vi "Run.vi"(8 "error in (no error)":errorcluster, 11 "Channel GUI in":refnum<class "Channel GEI.lvclass">) -> (0 "error out":errorcluster, 3 "Channel GUI out":refnum<class "Channel GEI.lvclass">)   [LabVIEW 2018, in "Channel GEI.lvclass"]
uses:
  Channel GEI.lvclass
  Channel GEI.lvclass/Channel GEI.ctl
  Interface/Interface.lvclass/Interface.ctl
  State Machine/State Machine.lvclass
  RxTx/RxTx.lvclass
  Interface/Interface.lvclass
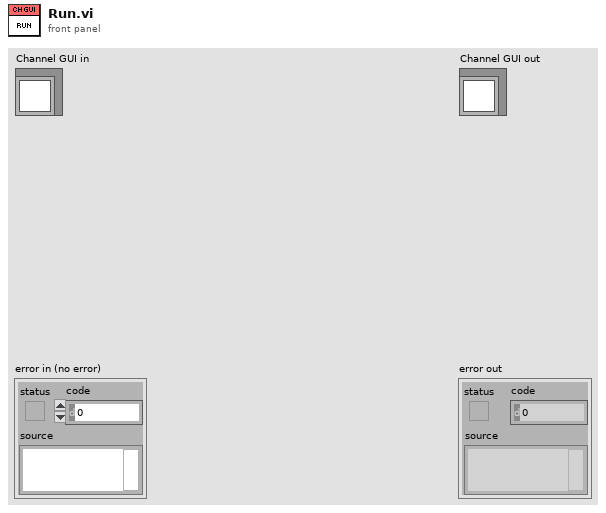
[diagram p1: front panel]
types:
  T1 = cluster{"COOLER_POWER_STATUS":u16, "TEMP":i32, "EXPTIME":dbl, "#FRAMES":u32, "#CUBES":u32}
  T2 = cluster{"CUBE_EXPOSURE_TIME":sgl, "CUBES_DONE":u16, "LAST_IMAGE_NAME":string, "DISK_SPACE":u16, "FRAMES_DONE":u16, "CCD_STATUS":string, "CURRENT_TEMPERATURE":i16, "TEMPERATURE_STATUS":string, "FRAME_EXPOSURE_TIME":u16, "CCD_ON_OFF":bool, "SERIAL_NUMBER":u16, "ACQUIRING":bool}
  T3 = cluster{"PREAMP":u16, "READOUT_RATE":u16, "EM_GAIN":u16, "VBIN":u16, "INITIAL_LINE":u16, "INITIAL_COLUMN":u16, "FINAL_LINE":u16, "FINAL_COLUMN":u16, "TRIGGER_MODE":u16, "HBIN":u16, "SHUTTER_TTL":u16, "SHUTTER_MODE":u16, "SHUTTER_OPENING_TIME":u16, "SHUTTER_CLOSING_TIME":u16, "VERTICAL_SHIFT_SPEED":u16, "READ_MODE":u16, "FRAME_TRANSFER":bool, "VERTICAL_CLOCK_VOLTAGE":u16, "ACQUISITION_MODE":u16, "AD_CHANNEL":u16, "EM_MODE":u16}
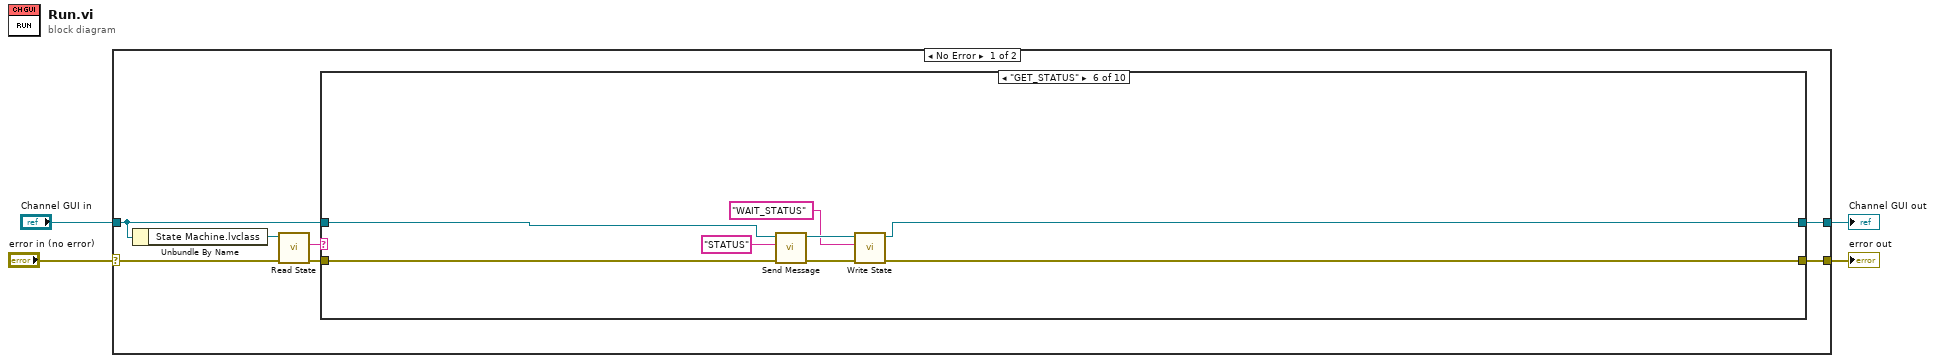
[diagram p0: block diagram]
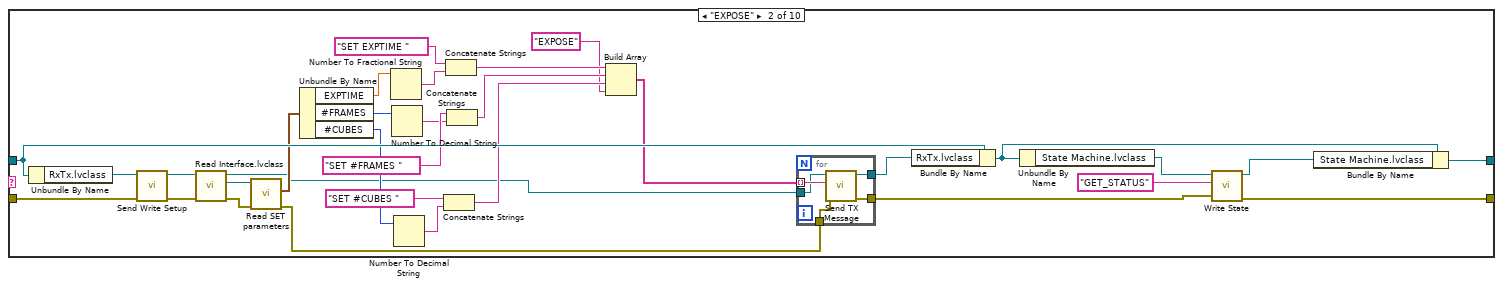
[diagram p3: hidden frame]
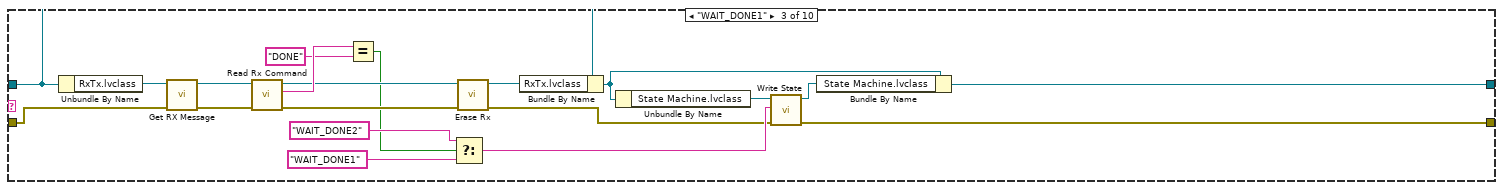
[diagram p4: hidden frame]
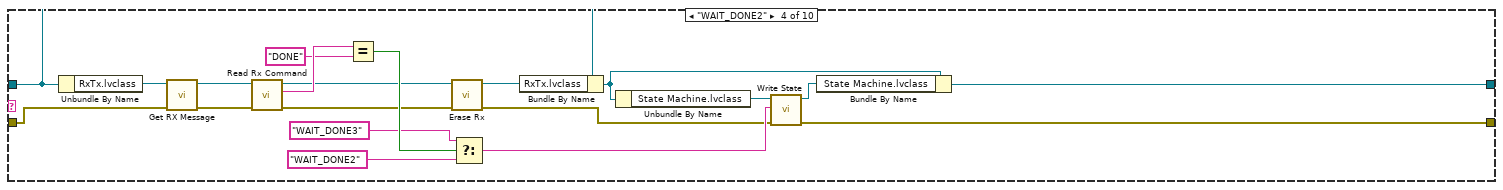
[diagram p5: hidden frame]
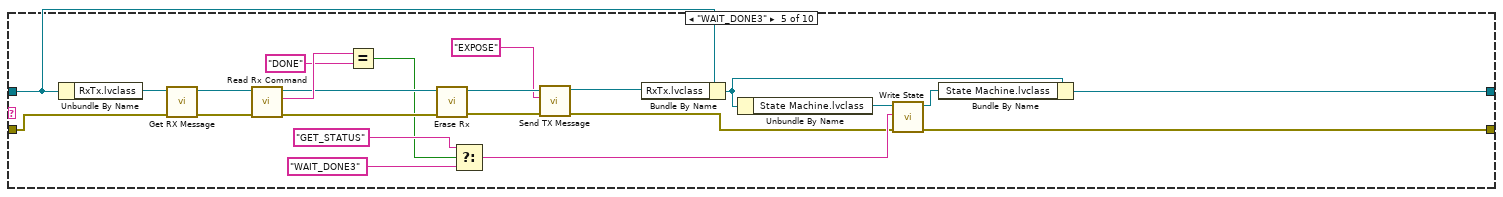
[diagram p6: hidden frame]
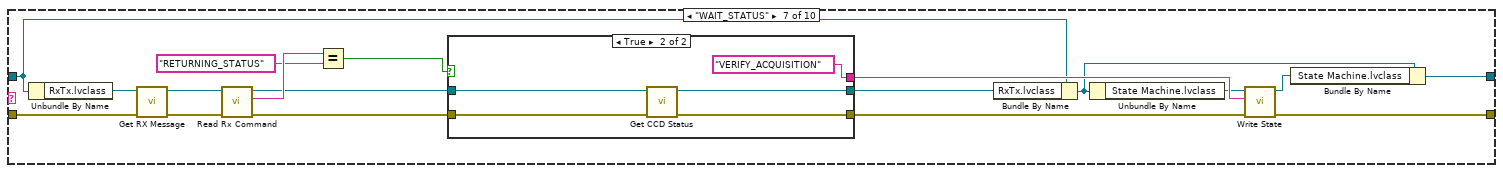
[diagram p7: hidden frame]
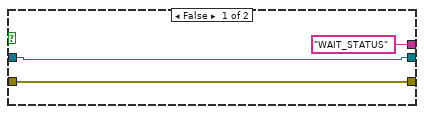
[diagram p8: hidden frame]
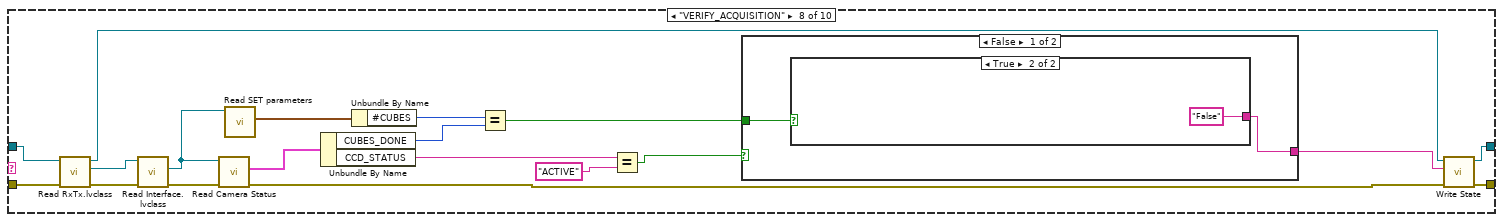
[diagram p9: hidden frame]
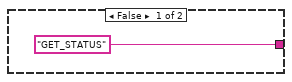
[diagram p10: hidden frame]
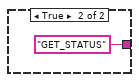
[diagram p11: hidden frame]
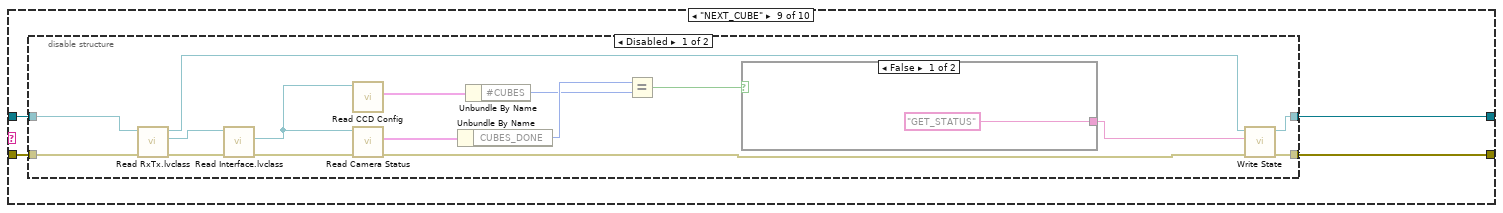
[diagram p12: hidden frame]
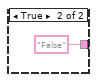
[diagram p13: hidden frame]
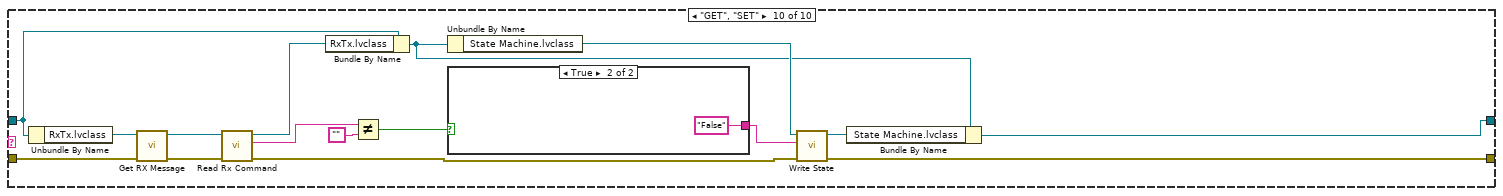
[diagram p15: hidden frame]
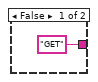
[diagram p16: hidden frame]
diagram:
  n1 = case shown="No Error" "error in (no error)" {
    selector: "error in (no error)" -> [w9 w215]
    tunnel: [w11 w215] -> w2
    tunnel: "Channel GUI in" -> [w7 w214]
    tunnel: [w6 w214] -> w1
    frame No Error {
      n2 = Unbundle By Name(w7) -> ("State Machine.lvclass"=w10:refnum<class "State Machine.lvclass">)
      n3 = call-dynamic "Read State.vi"("error in (no error)"=w9, "State Machine in"=w10) -> ("error out"=w8:errorcluster, "State"=w5:string)  [unwired: 7 in, 1 out]
      n4 = case shown="\"GET_STATUS\"" w5 {
        tunnel: w8 -> [w13 w37 w65 w85 w108 w121 w136 w159 w172 w208]
        tunnel: [w13 w41 w61 w81 w104 w116 w139 w165 w174 w211] -> w11
        tunnel: w7 -> [w12 w43 w60 w80 w103 w114 w125 w160 w173 w200]
        tunnel: [w12 w42 w62 w82 w105 w117 w123 w166 w175 w198] -> w6
        frame "False", Default {
        }
        frame "EXPOSE" {
          n5 = Unbundle By Name(w43) -> ("RxTx.lvclass"=w38:refnum<class "RxTx.lvclass">)
          n6 = call "Send Write Setup.vi"("error in (no error)"=w37, "RxTx in"=w38) -> ("error out"=w33:errorcluster, "RxTx out"=w34:refnum<class "RxTx.lvclass">)  [unwired: 8 in]
          n7 = call "Read Interface.lvclass.vi"("error in (no error)"=w33, "RxTx in"=w34) -> ("error out"=w31:errorcluster, "Interface.lvclass"=w32:refnum<class "Interface.lvclass">, "RxTx out"=w16:refnum<class "RxTx.lvclass">)  [unwired: 7 in]
          n8 = call "Read SET parameters.vi"("error in (no error)"=w31, "Interface in"=w32) -> ("error out"=w15:errorcluster, "SET parameters"=w29:T1)  [unwired: 7 in, 1 out]
          n9 = Unbundle By Name(w29) -> ("EXPTIME"=w28:dbl, "#FRAMES"=w26:u32, "#CUBES"=w21:u32)
          n10 = Number To Fractional String(number=w28) -> (F-format string=w30:string)  [unwired: 3 in]
          n11 = Number To Decimal String(number=w26) -> (decimal integer string=w24:string)  [unwired: 1 in]
          n12 = Number To Decimal String(number=w21) -> (decimal integer string=w22:string)  [unwired: 1 in]
          n13 = Concatenate Strings("SET #CUBES ", w22) -> (w18:string)
          n14 = Concatenate Strings("SET EXPTIME ", w30) -> (w20:string)
          n15 = Concatenate Strings("SET #FRAMES ", w24) -> (w19:string)
          n16 = Build Array(w20, w19, w18, "EXPOSE") -> (w17:string[])
          n17 = for {
            tunnel: [w50] -> w36
            tunnel: [w49] -> w35
            tunnel: w17 -> [w48] mode=indexing
            tunnel: w16 -> [w47]
            tunnel: w15 -> [w46]
            n18 = call "Send TX Message.vi"("error in (no error)"=w46, "element"=w48, "RxTx in"=w47) -> ("error out"=w50:errorcluster, "RxTx out"=w49:refnum<class "RxTx.lvclass">)  [unwired: 7 in]
          }
          n19 = Bundle By Name(cluster=w43, "RxTx.lvclass"=w35) -> (w44:refnum<class "Channel GEI.lvclass">)
          n20 = Unbundle By Name(w44) -> ("State Machine.lvclass"=w45:refnum<class "State Machine.lvclass">)
          n21 = call-dynamic "Write State.vi"("error in (no error)"=w36, "State"="GET_STATUS" ("New_State"), "State Machine in"=w45) -> ("error out"=w41:errorcluster, "State Machine out"=w40:refnum<class "State Machine.lvclass">)  [unwired: 7 in]
          n22 = Bundle By Name(cluster=w44, "State Machine.lvclass"=w40) -> (w42:refnum<class "Channel GEI.lvclass">)
        }
        frame "WAIT_DONE1" {
          n23 = Unbundle By Name(w60) -> ("RxTx.lvclass"=w70:refnum<class "RxTx.lvclass">)
          n24 = call "Get RX Message.vi"("error in (no error)"=w65, "RxTx in"=w70) -> ("error out"=w69:errorcluster, "RxTx out"=w68:refnum<class "RxTx.lvclass">)  [unwired: 8 in]
          n25 = call "Read Rx Command.vi"("error in (no error)"=w69, "RxTx in"=w68) -> ("error out"=w53:errorcluster, "Rx Command"=w67:string, "RxTx out"=w52:refnum<class "RxTx.lvclass">)  [unwired: 7 in]
          n26 = Equal?(x=w67, y="DONE") -> (x = y?=w51:bool)
          n27 = Select(t="WAIT_DONE2", s=w51, f="WAIT_DONE1") -> (s? t:f=w56:string)
          n28 = call "Erase Rx.vi"("error in (no error)"=w53, "RxTx in"=w52) -> ("error out"=w54:errorcluster, "RxTx out"=w55:refnum<class "RxTx.lvclass">)  [unwired: 8 in]
          n29 = Bundle By Name(cluster=w60, "RxTx.lvclass"=w55) -> (w63:refnum<class "Channel GEI.lvclass">)
          n30 = Unbundle By Name(w63) -> ("State Machine.lvclass"=w59:refnum<class "State Machine.lvclass">)
          n31 = call-dynamic "Write State.vi"("error in (no error)"=w54, "State"=w56, "State Machine in"=w59) -> ("error out"=w61:errorcluster, "State Machine out"=w64:refnum<class "State Machine.lvclass">)  [unwired: 7 in]
          n32 = Bundle By Name(cluster=w63, "State Machine.lvclass"=w64) -> (w62:refnum<class "Channel GEI.lvclass">)
        }
        frame "WAIT_DONE2" {
          n33 = Unbundle By Name(w80) -> ("RxTx.lvclass"=w90:refnum<class "RxTx.lvclass">)
          n34 = call "Get RX Message.vi"("error in (no error)"=w85, "RxTx in"=w90) -> ("error out"=w89:errorcluster, "RxTx out"=w88:refnum<class "RxTx.lvclass">)  [unwired: 8 in]
          n35 = call "Read Rx Command.vi"("error in (no error)"=w89, "RxTx in"=w88) -> ("error out"=w71:errorcluster, "Rx Command"=w87:string, "RxTx out"=w72:refnum<class "RxTx.lvclass">)  [unwired: 7 in]
          n36 = Equal?(x=w87, y="DONE") -> (x = y?=w78:bool)
          n37 = call "Erase Rx.vi"("error in (no error)"=w71, "RxTx in"=w72) -> ("error out"=w73:errorcluster, "RxTx out"=w74:refnum<class "RxTx.lvclass">)  [unwired: 8 in]
          n38 = Select(t="WAIT_DONE3", s=w78, f="WAIT_DONE2") -> (s? t:f=w75:string)
          n39 = Bundle By Name(cluster=w80, "RxTx.lvclass"=w74) -> (w83:refnum<class "Channel GEI.lvclass">)
          n40 = Unbundle By Name(w83) -> ("State Machine.lvclass"=w79:refnum<class "State Machine.lvclass">)
          n41 = call-dynamic "Write State.vi"("error in (no error)"=w73, "State"=w75, "State Machine in"=w79) -> ("error out"=w81:errorcluster, "State Machine out"=w84:refnum<class "State Machine.lvclass">)  [unwired: 7 in]
          n42 = Bundle By Name(cluster=w83, "State Machine.lvclass"=w84) -> (w82:refnum<class "Channel GEI.lvclass">)
        }
        frame "WAIT_DONE3" {
          n43 = Unbundle By Name(w103) -> ("RxTx.lvclass"=w113:refnum<class "RxTx.lvclass">)
          n44 = call "Get RX Message.vi"("error in (no error)"=w108, "RxTx in"=w113) -> ("error out"=w112:errorcluster, "RxTx out"=w111:refnum<class "RxTx.lvclass">)  [unwired: 8 in]
          n45 = call "Read Rx Command.vi"("error in (no error)"=w112, "RxTx in"=w111) -> ("error out"=w97:errorcluster, "Rx Command"=w110:string, "RxTx out"=w98:refnum<class "RxTx.lvclass">)  [unwired: 7 in]
          n46 = Equal?(x=w110, y="DONE") -> (x = y?=w96:bool)
          n47 = call "Erase Rx.vi"("error in (no error)"=w97, "RxTx in"=w98) -> ("error out"=w92:errorcluster, "RxTx out"=w95:refnum<class "RxTx.lvclass">)  [unwired: 8 in]
          n48 = Select(t="GET_STATUS", s=w96, f="WAIT_DONE3") -> (s? t:f=w99:string)
          n49 = call "Send TX Message.vi"("error in (no error)"=w92, "element"="EXPOSE", "RxTx in"=w95) -> ("error out"=w93:errorcluster, "RxTx out"=w94:refnum<class "RxTx.lvclass">)  [unwired: 7 in]
          n50 = Bundle By Name(cluster=w103, "RxTx.lvclass"=w94) -> (w106:refnum<class "Channel GEI.lvclass">)
          n51 = Unbundle By Name(w106) -> ("State Machine.lvclass"=w102:refnum<class "State Machine.lvclass">)
          n52 = call-dynamic "Write State.vi"("error in (no error)"=w93, "State"=w99, "State Machine in"=w102) -> ("error out"=w104:errorcluster, "State Machine out"=w107:refnum<class "State Machine.lvclass">)  [unwired: 7 in]
          n53 = Bundle By Name(cluster=w106, "State Machine.lvclass"=w107) -> (w105:refnum<class "Channel GEI.lvclass">)
        }
        frame "GET_STATUS" {
          n54 = call "Send Message.vi"("error in (no error)"=w121, "Message"="STATUS", "Channel GUI in"=w114) -> ("error out"=w119:errorcluster, "Channel GUI out"=w118:refnum<class "Channel GEI.lvclass">)  [unwired: 7 in]
          n55 = call "Write State.vi"("error in (no error)"=w119, "State"="WAIT_STATUS" ("Message"), "Channel GEI in"=w118) -> ("error out"=w116:errorcluster, "Channel GEI out"=w117:refnum<class "Channel GEI.lvclass">)  [unwired: 7 in]
        }
        frame "WAIT_STATUS" {
          n56 = Unbundle By Name(w125) -> ("RxTx.lvclass"=w137:refnum<class "RxTx.lvclass">)
          n57 = call "Get RX Message.vi"("error in (no error)"=w136, "RxTx in"=w137) -> ("error out"=w135:errorcluster, "RxTx out"=w134:refnum<class "RxTx.lvclass">)  [unwired: 8 in]
          n58 = call "Read Rx Command.vi"("error in (no error)"=w135, "RxTx in"=w134) -> ("error out"=w130:errorcluster, "Rx Command"=w131:string, "RxTx out"=w129:refnum<class "RxTx.lvclass">)  [unwired: 7 in]
          n59 = Equal?(x=w131, y="RETURNING_STATUS") -> (x = y?=w132:bool)
          n60 = case shown="True" w132 {
            tunnel: ["WAIT_STATUS" "VERIFY_ACQUISITION"] -> w133
            tunnel: w130 -> [w140 w146]
            tunnel: w129 -> [w141 w145]
            tunnel: [w140 w144] -> w128
            tunnel: [w141 w143] -> w127
            frame False {
            }
            frame True {
              n61 = call "Get CCD Status.vi"("error in (no error)"=w146, "RxTx in"=w145) -> ("error out"=w144:errorcluster, "RxTx out"=w143:refnum<class "RxTx.lvclass">)  [unwired: 8 in]
            }
          }
          n62 = Bundle By Name(cluster=w125, "RxTx.lvclass"=w127) -> (w124:refnum<class "Channel GEI.lvclass">)
          n63 = Unbundle By Name(w124) -> ("State Machine.lvclass"=w126:refnum<class "State Machine.lvclass">)
          n64 = call-dynamic "Write State.vi"("error in (no error)"=w128, "State"=w133, "State Machine in"=w126) -> ("error out"=w139:errorcluster, "State Machine out"=w138:refnum<class "State Machine.lvclass">)  [unwired: 7 in]
          n65 = Bundle By Name(cluster=w124, "State Machine.lvclass"=w138) -> (w123:refnum<class "Channel GEI.lvclass">)
        }
        frame "VERIFY_ACQUISITION" {
          n66 = call "Read RxTx.lvclass.vi"("error in (no error)"=w159, "Channel GUI in"=w160) -> ("error out"=w163:errorcluster, "RxTx.lvclass"=w161:refnum<class "RxTx.lvclass">, "Channel GUI out"=w154:refnum<class "Channel GEI.lvclass">)  [unwired: 7 in]
          n67 = call "Read Interface.lvclass.vi"("error in (no error)"=w163, "RxTx in"=w161) -> ("error out"=w162:errorcluster, "Interface.lvclass"=w150:refnum<class "Interface.lvclass">)  [unwired: 7 in, 1 out]
          n68 = call "Read Camera Status.vi"("error in (no error)"=w162, "Interface in"=w150) -> ("error out"=w153:errorcluster, "Camera Status"=w158:T2)  [unwired: 7 in, 1 out]
          n69 = call "Read SET parameters.vi"("Interface in"=w150) -> ("SET parameters"=w149:T1)  [unwired: 8 in, 2 out]
          n70 = Unbundle By Name(w158) -> ("CUBES_DONE"=w152:u16, "CCD_STATUS"=w157:string)
          n71 = Unbundle By Name(w149) -> ("#CUBES"=w148:u32)
          n72 = Equal?(x=w148, y=w152) -> (x = y?=w151:bool)
          n73 = Equal?(x=w157, y="ACTIVE" ("Message")) -> (x = y?=w155:bool)
          n74 = case shown="False" w155 {
            tunnel: [w168 "GET_STATUS" ("Message")] -> w164
            tunnel: w151 -> [w167 _]
            frame False {
              n75 = case shown="True" w167 {
                tunnel: ["GET_STATUS" ("Message") "False" ("Message")] -> w168
                frame False {
                }
                frame True {
                }
              }
            }
            frame True {
            }
          }
          n76 = call "Write State.vi"("error in (no error)"=w153, "State"=w164, "Channel GEI in"=w154) -> ("error out"=w165:errorcluster, "Channel GEI out"=w166:refnum<class "Channel GEI.lvclass">)  [unwired: 7 in]
        }
        frame "NEXT_CUBE" {
          n77 = disable-structure shown="Disabled" {
            disable-tunnel: [w191 w195] -> w175
            disable-tunnel: [w190 w194] -> w174
            disable-tunnel: w173 -> [w185 w195]
            disable-tunnel: w172 -> [w184 w194]
            frame Disabled {
              n78 = call "Read RxTx.lvclass.vi"("error in (no error)"=w184, "Channel GUI in"=w185) -> ("error out"=w188:errorcluster, "RxTx.lvclass"=w186:refnum<class "RxTx.lvclass">, "Channel GUI out"=w180:refnum<class "Channel GEI.lvclass">)  [unwired: 7 in]
              n79 = call "Read Interface.lvclass.vi"("error in (no error)"=w188, "RxTx in"=w186) -> ("error out"=w187:errorcluster, "Interface.lvclass"=w178:refnum<class "Interface.lvclass">)  [unwired: 7 in, 1 out]
              n80 = call "Read CCD Config.vi"("Interface in"=w178) -> ("Previous CCD Config"=w177:T3)  [unwired: 8 in, 2 out]
              n81 = call "Read Camera Status.vi"("error in (no error)"=w187, "Interface in"=w178) -> ("error out"=w179:errorcluster, "Camera Status"=w183:T2)  [unwired: 7 in, 1 out]
              n82 = Unbundle By Name(w183) -> ("CUBES_DONE"=w182:u16)
              n83 = Unbundle By Name(w177) -> ("#CUBES"=w176:u32)
              n84 = Equal?(x=w182, y=w176) -> (x = y?=w181:bool)
              n85 = case shown="False" w181 {
                tunnel: ["GET_STATUS" ("Message") "False" ("Message")] -> w189
                frame False {
                }
                frame True {
                }
              }
              n86 = call "Write State.vi"("error in (no error)"=w179, "State"=w189, "Channel GEI in"=w180) -> ("error out"=w190:errorcluster, "Channel GEI out"=w191:refnum<class "Channel GEI.lvclass">)  [unwired: 7 in]
            }
            frame Enabled {
            }
          }
        }
        frame "GET", "SET" {
          n87 = Unbundle By Name(w200) -> ("RxTx.lvclass"=w209:refnum<class "RxTx.lvclass">)
          n88 = call "Get RX Message.vi"("error in (no error)"=w208, "RxTx in"=w209) -> ("error out"=w207:errorcluster, "RxTx out"=w206:refnum<class "RxTx.lvclass">)  [unwired: 8 in]
          n89 = call "Read Rx Command.vi"("error in (no error)"=w207, "RxTx in"=w206) -> ("error out"=w196:errorcluster, "Rx Command"=w202:string, "RxTx out"=w197:refnum<class "RxTx.lvclass">)  [unwired: 7 in]
          n90 = Bundle By Name(cluster=w200, "RxTx.lvclass"=w197) -> (w199:refnum<class "Channel GEI.lvclass">)
          n91 = Not Equal?(x=w202, y="") -> (x != y?=w204:bool)
          n92 = Unbundle By Name(w199) -> ("State Machine.lvclass"=w201:refnum<class "State Machine.lvclass">)
          n93 = case shown="True" w204 {
            tunnel: ["GET" "False"] -> w205
            frame False {
            }
            frame True {
            }
          }
          n94 = call-dynamic "Write State.vi"("error in (no error)"=w196, "State"=w205, "State Machine in"=w201) -> ("error out"=w211:errorcluster, "State Machine out"=w210:refnum<class "State Machine.lvclass">)  [unwired: 7 in]
          n95 = Bundle By Name(cluster=w199, "State Machine.lvclass"=w210) -> (w198:refnum<class "Channel GEI.lvclass">)
        }
      }
    }
    frame Error {
    }
  }
  "error out" <- w2
  "Channel GUI out" <- w1
